vi "picoharp_process_records.vi"(8 "error in (no error)":errorcluster, 11 "hydraharp in":refnum<class "picoharp.lvclass">) -> (0 "error out":errorcluster, 3 "hydraharp out":refnum<class "picoharp.lvclass">)   [LabVIEW 2015, in "picoharp.lvclass"]
uses:
  picoharp.lvclass
  picoharp.lvclass/picoharp.ctl
  Data Logger Class/data_logger.lvclass
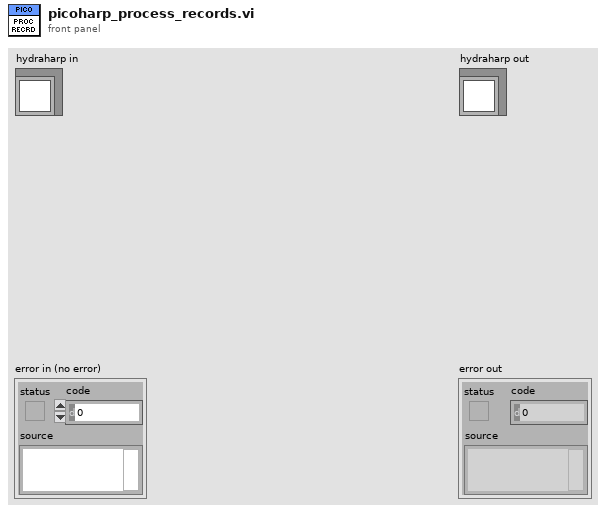
[diagram p1: front panel]
types:
  T1 = typedef "hydraharp_action_on_records.ctl" = enum16{"stream_to_file", "correlate", "stream to file and correlate", "histogram"}
  T2 = typedef "record_type.ctl" = enum16{"Raw Stream", "Processed Records (hdf5)"}
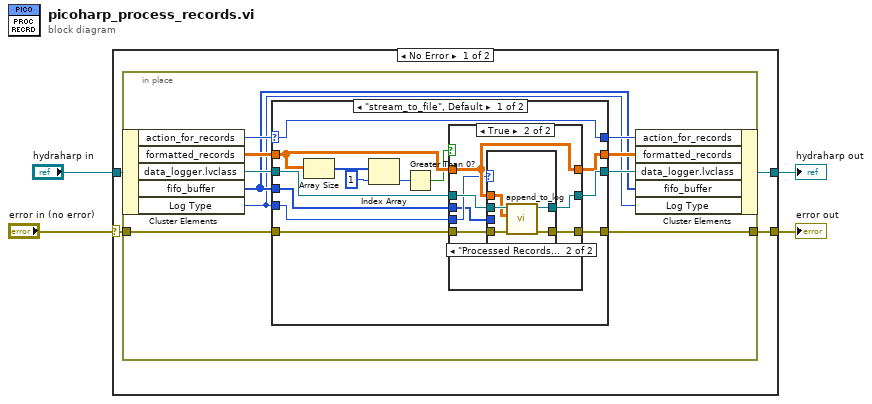
[diagram p0: block diagram]
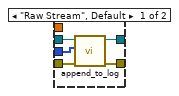
[diagram p3: hidden frame]
diagram:
  n1 = case shown="No Error" "error in (no error)" {
    selector: "error in (no error)" -> [w7 w57]
    tunnel: [w6 w57] -> w3
    tunnel: [w5 w56] -> w1
    tunnel: "hydraharp in" -> [w8 w56]
    frame No Error {
      n2 = in-place {
        in-place-border: w7 -> [w16]
        in-place-border: [w15] -> w6
        n3 = in-place-cluster #1(w8) -> ("action_for_records"=w18:T1, "formatted_records"=w17:dbl[][], "data_logger.lvclass"=w13:refnum<class "data_logger.lvclass">, "fifo_buffer"=w10:u32[], "Log Type"=w9:T2)
        n4 = case shown="\"stream_to_file\", Default" w18 {
          selector: w18 -> [w31 w55]
          tunnel: w17 -> [w28 w52]
          tunnel: w16 -> [w30 w54]
          tunnel: [w29 w54] -> w15
          tunnel: [w31 w55] -> w14
          tunnel: w13 -> [w23 w53]
          tunnel: [w22 w53] -> w12
          tunnel: [w21 w52] -> w11
          tunnel: w9 -> [w20 _]
          tunnel: w10 -> [w19 _]
          frame "stream_to_file", Default {
            n5 = Array Size(array=w28) -> (size(s)=w27:i32[])
            n6 = Index Array(array=w27, index=1) -> (element=w25:i32)
            n7 = Greater Than 0?(x=w25) -> (x > 0?=w24:bool)
            n8 = case shown="True" w24 {
              tunnel: w30 -> [w34 w41]
              tunnel: [w34 w40] -> w29
              tunnel: w28 -> [w32 w37]
              tunnel: w23 -> [w33 w39]
              tunnel: [w33 w38] -> w22
              tunnel: [w32 w37] -> w21
              tunnel: w20 -> [_ w36]
              tunnel: w19 -> [_ w35]
              frame False {
              }
              frame True {
                n9 = case shown="\"Processed Records (hdf5)\"" w36 {
                  tunnel: w41 -> [w43 w51]
                  tunnel: [w44 w50] -> w40
                  tunnel: w39 -> [w46 w49]
                  tunnel: [w45 w48] -> w38
                  tunnel: w37 -> [_ w47]
                  tunnel: w35 -> [w42 _]
                  frame "Raw Stream", Default {
                    n10 = call-dynamic "append_to_log.vi"("error in (no error)"=w43, "Data"=w42, "data_logger in"=w46) -> ("error out"=w44:errorcluster, "data_logger out"=w45:refnum<class "data_logger.lvclass">)  [unwired: 7 in]
                  }
                  frame "Processed Records (hdf5)" {
                    n11 = call-dynamic "append_to_log.vi"("error in (no error)"=w51, "Data"=w47, "data_logger in"=w49) -> ("error out"=w50:errorcluster, "data_logger out"=w48:refnum<class "data_logger.lvclass">)  [unwired: 7 in]
                  }
                }
              }
            }
          }
          frame "correlate" {
          }
        }
        n12 = in-place-cluster #1("action_for_records"=w14, "formatted_records"=w11, "data_logger.lvclass"=w12, "fifo_buffer"=w10, "Log Type"=w9) -> (w5:refnum<class "picoharp.lvclass">)
      }
    }
    frame Error {
    }
  }
  "error out" <- w3
  "hydraharp out" <- w1
